vi "getFPimage.vi"(7 "LabVIEW Web Service Request":refnum<class "Web Request.lvclass">) -> ()   [LabVIEW 2014]
uses:
  <vilib>/wsapi/Web Request.lvclass
panel:
  # "Use the Web Service Request input terminal to call the VIs on the Web Services palette. Do not remove it from the connector pane unless you don't need access to the palette."
  # "Each additional control wired to the connector pane will be available as an input in the URL. To include an indicator in terminal-mode output (the default setting), it must also be wired to the connector pane."
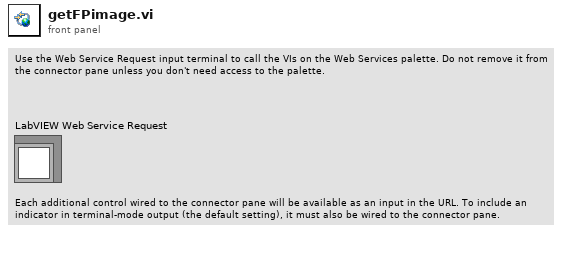
[diagram p1: front panel]
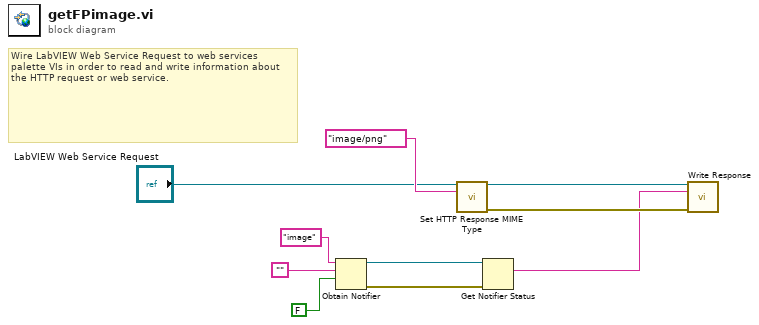
[diagram p0: block diagram]
diagram:
  # "Wire LabVIEW Web Service Request to web services palette VIs in order to read and write information about the HTTP request or web service."
  n1 = Obtain Notifier(name (unnamed)="image", notification data type="", create if not found? (T)=FALSE) -> (notifier out=w8:refnum<notifier>, error out=w7:errorcluster)  [unwired: 1 in, 1 out]
  n2 = call <vilib>:"Set HTTP Response MIME Type.vi"("LabVIEW Web Service Request"="LabVIEW Web Service Request", "MIME type (text/html)"="image/png") -> ("LabVIEW Web Service Request out"=w4:refnum<class "Web Request.lvclass">, "error out"=w3:errorcluster)  [unwired: 12 in]
  n3 = Get Notifier Status(notifier=w8, error in (no error)=w7) -> (current notification=w1:string)  [unwired: 4 out]
  n4 = call <vilib>:"Write Response.vi"("LabVIEW Web Service Request"=w4, "response string"=w1, "error in (no error)"=w3) -> ()  [unwired: 11 in, 2 out]
